vi "CheckForDeath.vi"(8 "error in (no error)":errorcluster, 10 "BlockedSpots":T1[](array[typedef]), 11 "Snake in":refnum<class "Snake.lvclass">) -> (0 "error out":errorcluster, 3 "Snake out":refnum<class "Snake.lvclass">)   [LabVIEW 2019, in "RT_Game.lvlib" / "Snake.lvclass"]
uses:
  Snake.lvclass
  Game/Coordinate.ctl
  Snake.lvclass/Snake.ctl
  Game/Game.lvclass
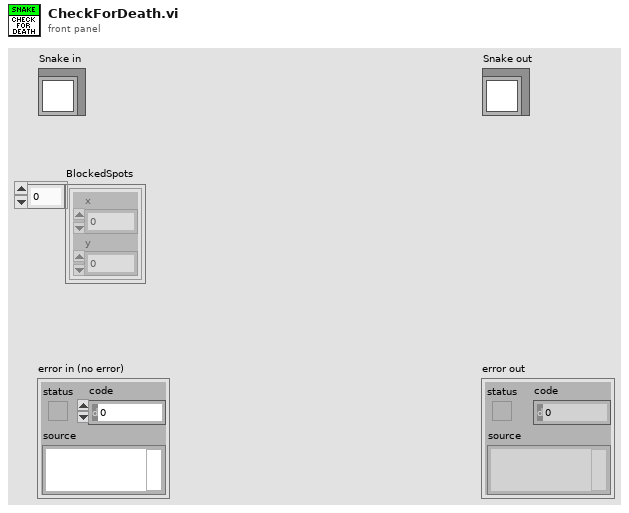
[diagram p1: front panel]
types:
  T1 = typedef "RT_Game.lvlib/Game.lvclass/Coordinate.ctl" = cluster{"x":dbl, "y":dbl}
  T2 = typedef "RT_Game.lvlib/SnakeGame.lvclass/CoordinateData.ctl" = cluster{"Coordinate":T1, "TileCode":u16}
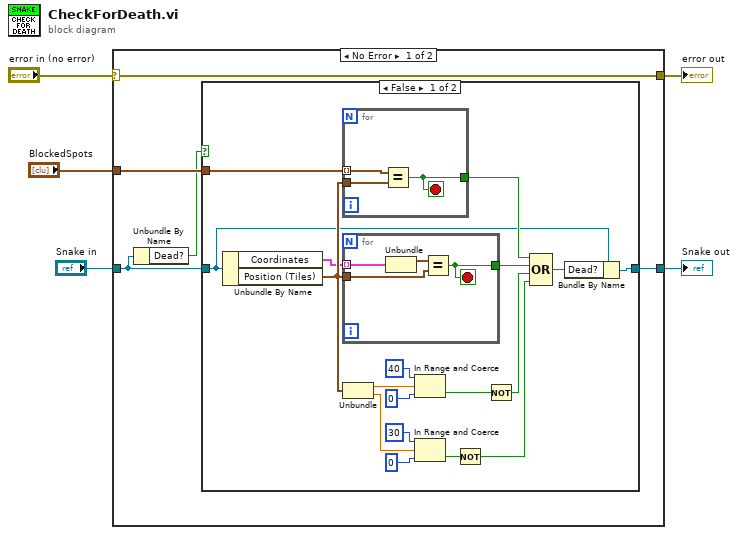
[diagram p0: block diagram]
diagram:
  n1 = case shown="No Error" "error in (no error)" {
    selector: "error in (no error)" -> [w10 w38]
    tunnel: [w10 w38] -> w4
    tunnel: [w7 w37] -> w2
    tunnel: "Snake in" -> [w9 w37]
    tunnel: "BlockedSpots" -> [w8 _]
    frame No Error {
      n2 = Unbundle By Name(w9) -> ("Dead?"=w6:bool)
      n3 = case shown="False" w6 {
        tunnel: w9 -> [w14 w36]
        tunnel: w8 -> [w13 _]
        tunnel: [w12 w36] -> w7
        frame False {
          n4 = Unbundle By Name(w14) -> ("Coordinates"=w15:T2[], "Position (Tiles)"=w27:T1)
          n5 = for {
            tunnel: w13 -> [w29] mode=indexing
            tunnel: w27 -> [w31]
            tunnel: [w30] -> w28
            stop <- w30 stop-if-true
            n6 = Equal?(x=w29, y=w31) -> (x = y?=w30:bool)
          }
          n7 = for {
            tunnel: w15 -> [w34] mode=indexing
            tunnel: w27 -> [w35]
            tunnel: [w33] -> w16
            stop <- w33 stop-if-true
            n8 = Unbundle(w34) -> ("Coordinate"=w32:T1)  [unwired: 1 out]
            n9 = Equal?(x=w32, y=w35) -> (x = y?=w33:bool)
          }
          n10 = Unbundle(w27) -> ("x"=w17:dbl, "y"=w20:dbl)
          n11 = In Range and Coerce(upper limit=i8 40, x=w17, lower limit=i8 0) -> (In Range?=w23:bool)  [unwired: 1 out]
          n12 = In Range and Coerce(upper limit=i8 30, x=w20, lower limit=i8 0) -> (In Range?=w24:bool)  [unwired: 1 out]
          n13 = Not(x=w24) -> (.not. x?=w26:bool)
          n14 = Not(x=w23) -> (.not. x?=w25:bool)
          n15 = Compound Arithmetic op=OR(w28, w16, w25, w26) -> (w11:bool)
          n16 = Bundle By Name(cluster=w14, "Dead?"=w11) -> (w12:refnum<class "Snake.lvclass">)
        }
        frame True {
        }
      }
    }
    frame Error {
    }
  }
  "error out" <- w4
  "Snake out" <- w2
